vi "Self Event.vi"(9 "Priority?":bool, 10 "Msg Strategy":refnum<class "Msg Strategy.lvclass">, 11 "Hello World Event in":refnum<class "Hello World Event.lvclass">) -> (3 "Hello World Event out":refnum<class "Hello World Event.lvclass">)   [LabVIEW 2021, in "Hello World Event.lvlib" / "Hello World Event.lvclass"]
uses:
  Hello World Event.lvclass
  jettl/Msg Strategy/Msg Strategy.lvclass
  Hello World Event.lvclass/Hello World Event.ctl
  jettl/Event/Event.lvclass
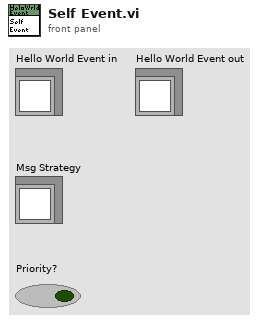
[diagram p1: front panel]
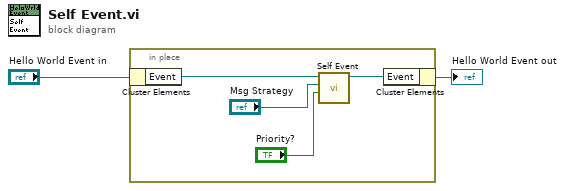
[diagram p0: block diagram]
diagram:
  n1 = in-place {
    n2 = in-place-cluster #1("Hello World Event in") -> ("Event"=w6:refnum<class "Event.lvclass">)
    n3 = call-dynamic "Self Event.vi"("Priority?"="Priority?", "Msg Strategy"="Msg Strategy", "Event in"=w6) -> ("Event out"=w5:refnum<class "Event.lvclass">)  [unwired: 8 in]
    n4 = in-place-cluster #1("Event"=w5) -> (→"Hello World Event out":refnum<class "Hello World Event.lvclass">)
  }
